vi "走到地.vi"(0 "房子數量":dbl, 1 "自己的地?":bool, 2 "旅館數量":dbl, 3 "編號":dbl, 4 "走到人財產":dbl) -> (5 "走到人-?":dbl, 6 "蓋第幾棟":dbl, 7 "地主+?":dbl, 8 "破產?":bool)   [LabVIEW 2014]
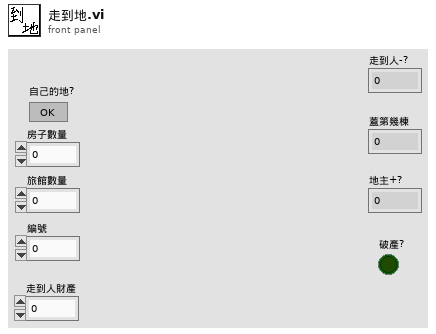
[diagram p1: front panel]
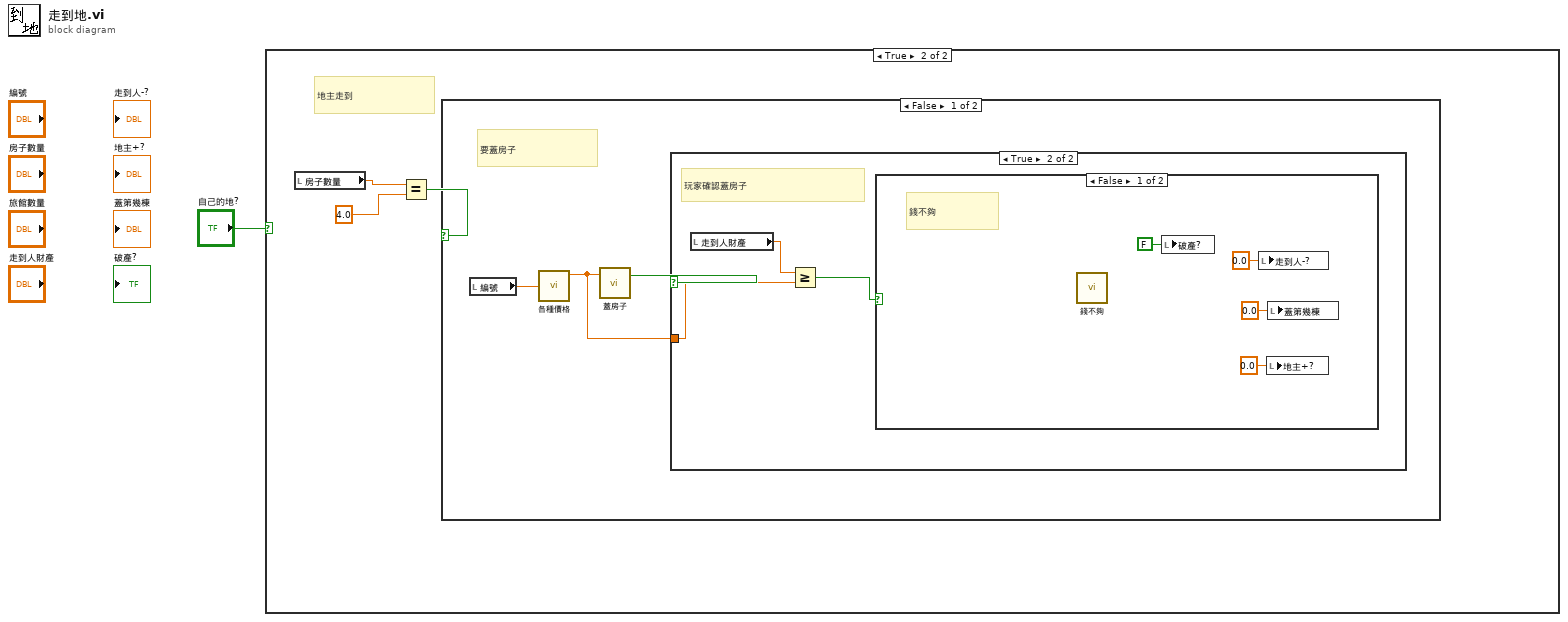
[diagram p0: block diagram]
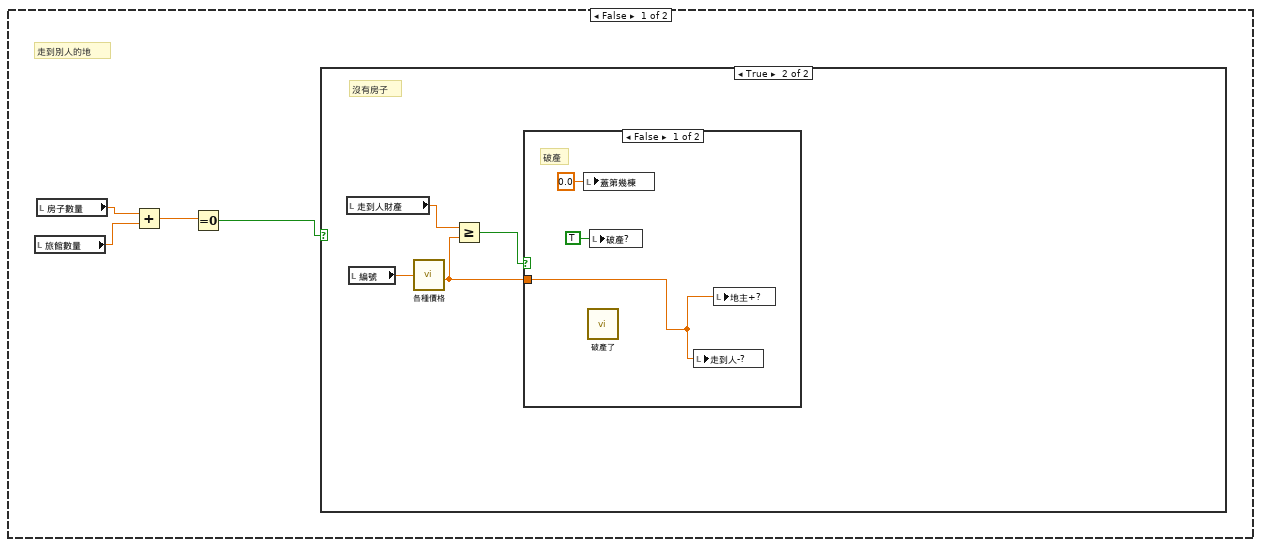
[diagram p2: hidden frame]
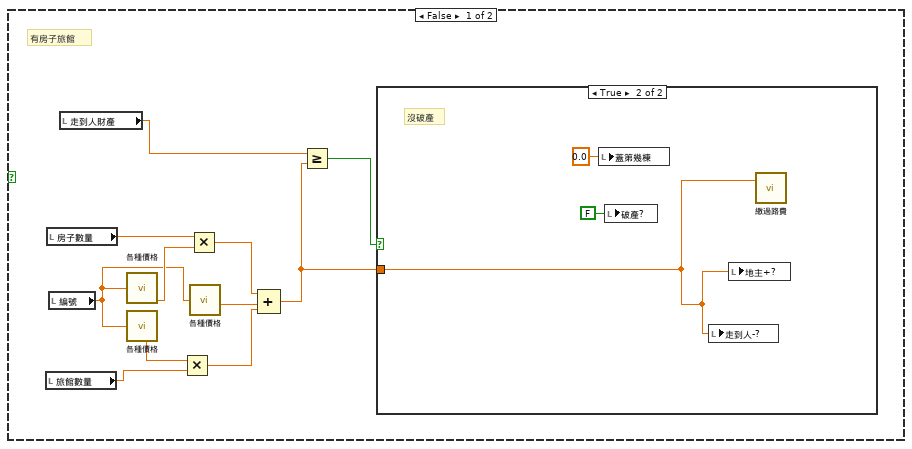
[diagram p3: hidden frame]
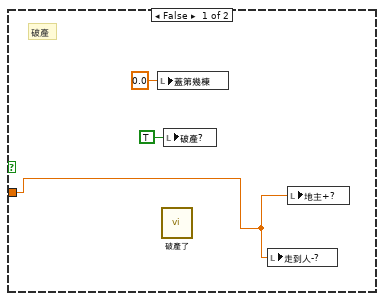
[diagram p4: hidden frame]
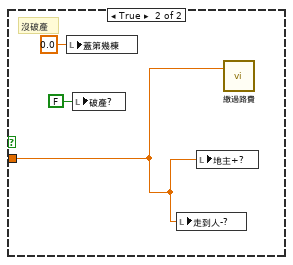
[diagram p5: hidden frame]
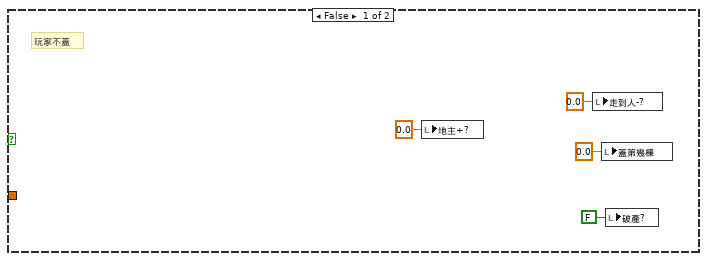
[diagram p6: hidden frame]
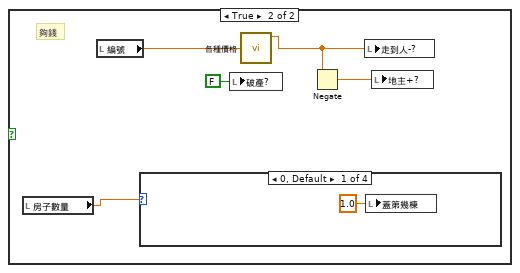
[diagram p7: hidden frame]
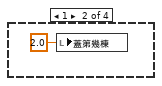
[diagram p8: hidden frame]
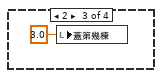
[diagram p9: hidden frame]
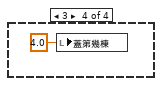
[diagram p10: hidden frame]
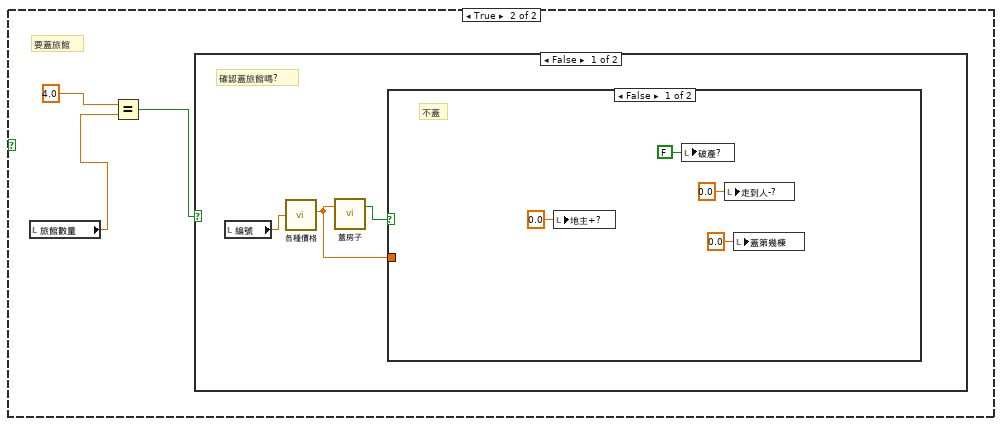
[diagram p11: hidden frame]
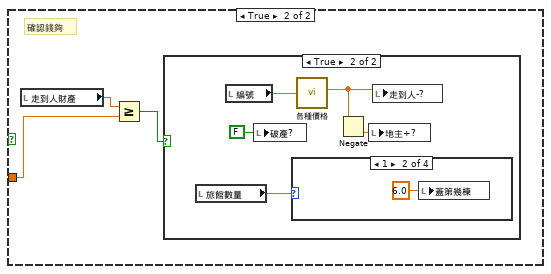
[diagram p12: hidden frame]
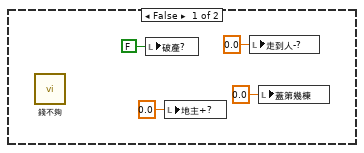
[diagram p13: hidden frame]
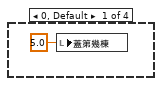
[diagram p14: hidden frame]
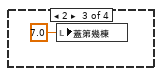
[diagram p15: hidden frame]
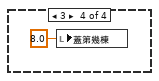
[diagram p16: hidden frame]
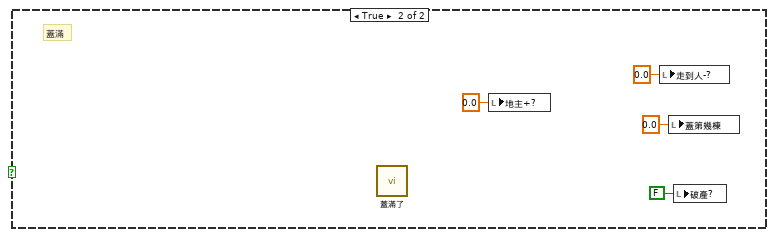
[diagram p17: hidden frame]
diagram:
  n1 = case shown="True" "自己的地?" {
    frame False {
      # "走到別人的地"
      n2 = local read "旅館數量"() -> (w4:dbl)
      n3 = local read "房子數量"() -> (w5:dbl)
      n4 = Add(x=w5, y=w4) -> (x+y=w3:dbl)
      n5 = Equal To 0?(x=w3) -> (x = 0?=w2:bool)
      n6 = case shown="True" w2 {
        frame False {
          # "有房子旅館"
          n7 = local read "旅館數量"() -> (w13:dbl)
          n8 = local read "房子數量"() -> (w16:dbl)
          n9 = local read "編號"() -> (w9:dbl)
          n10 = local read "走到人財產"() -> (w12:dbl)
          n11 = call "各種價格.vi"("Numeric"=w9) -> ("1房子費"=w15:dbl)  [unwired: 4 in, 5 out]
          n12 = call "各種價格.vi"("Numeric"=w9) -> ("1旅館費"=w14:dbl)  [unwired: 4 in, 5 out]
          n13 = Multiply(x=w14, y=w13) -> (x*y=w6:dbl)
          n14 = Multiply(x=w16, y=w15) -> (x*y=w7:dbl)
          n15 = call "各種價格.vi"("Numeric"=w9) -> ("空地費"=w8:dbl)  [unwired: 4 in, 5 out]
          n16 = Compound Arithmetic op=ADD(w7, w8, w6) -> (w10:dbl)
          n17 = Greater Or Equal?(x=w12, y=w10) -> (x >= y?=w11:bool)
          n18 = case shown="True" w11 {
            tunnel: w10 -> [w17 w20]
            frame False {
              # "破產"
              n19 = local write "蓋第幾棟"(0.0 ("蓋第幾棟")) -> ()
              n20 = call "破產了.vi"() -> ()  [unwired: 4 in]
              n21 = local write "破產?"(TRUE ("破產?")) -> ()
              n22 = local write "走到人-?"(w17) -> ()
              n23 = local write "地主+?"(w17) -> ()
            }
            frame True {
              # "沒破產"
              n24 = local write "蓋第幾棟"(0.0 ("蓋第幾棟")) -> ()
              n25 = local write "破產?"(FALSE ("破產?")) -> ()
              n26 = local write "走到人-?"(w20) -> ()
              n27 = local write "地主+?"(w20) -> ()
              n28 = call "繳過路費.vi"("過路費"=w20) -> ()  [unwired: 3 in]
            }
          }
        }
        frame True {
          # "沒有房子"
          n29 = local read "走到人財產"() -> (w25:dbl)
          n30 = local read "編號"() -> (w26:dbl)
          n31 = call "各種價格.vi"("Numeric"=w26) -> ("空地費"=w23:dbl)  [unwired: 4 in, 5 out]
          n32 = Greater Or Equal?(x=w25, y=w23) -> (x >= y?=w24:bool)
          n33 = case shown="False" w24 {
            tunnel: w23 -> [w27 w30]
            frame False {
              # "破產"
              n34 = local write "蓋第幾棟"(0.0 ("蓋第幾棟")) -> ()
              n35 = call "破產了.vi"() -> ()  [unwired: 4 in]
              n36 = local write "破產?"(TRUE ("破產?")) -> ()
              n37 = local write "走到人-?"(w27) -> ()
              n38 = local write "地主+?"(w27) -> ()
            }
            frame True {
              # "沒破產"
              n39 = local write "蓋第幾棟"(0.0 ("蓋第幾棟")) -> ()
              n40 = local write "破產?"(FALSE ("破產?")) -> ()
              n41 = local write "走到人-?"(w30) -> ()
              n42 = local write "地主+?"(w30) -> ()
              n43 = call "繳過路費.vi"("過路費"=w30) -> ()  [unwired: 3 in]
            }
          }
        }
      }
    }
    frame True {
      # "地主走到"
      n44 = local read "房子數量"() -> (w35:dbl)
      n45 = Equal?(x=w35, y=4.0) -> (x = y?=w33:bool)
      n46 = case shown="False" w33 {
        frame False {
          # "要蓋房子"
          n47 = local read "編號"() -> (w38:dbl)
          n48 = call "各種價格.vi"("Numeric"=w38) -> ("蓋房子"=w36:dbl)  [unwired: 4 in, 5 out]
          n49 = call "蓋房子.vi"("花費金額"=w36) -> ("確定 2"=w37:bool)  [unwired: 2 in]
          n50 = case shown="True" w37 {
            tunnel: w36 -> [_ w44]
            frame False {
              # "玩家不蓋"
              n51 = local write "地主+?"(0.0 ("地主+?")) -> ()
              n52 = local write "走到人-?"(0.0 ("走到人-?")) -> ()
              n53 = local write "蓋第幾棟"(0.0 ("蓋第幾棟")) -> ()
              n54 = local write "破產?"(FALSE ("破產?")) -> ()
            }
            frame True {
              # "玩家確認蓋房子"
              n55 = local read "走到人財產"() -> (w45:dbl)
              n56 = Greater Or Equal?(x=w45, y=w44) -> (x >= y?=w43:bool)
              n57 = case shown="False" w43 {
                frame False {
                  # "錢不夠"
                  n58 = call "錢不夠.vi"() -> ()  [unwired: 4 in]
                  n59 = local write "破產?"(FALSE ("破產?")) -> ()
                  n60 = local write "走到人-?"(0.0 ("走到人-?")) -> ()
                  n61 = local write "地主+?"(0.0 ("地主+?")) -> ()
                  n62 = local write "蓋第幾棟"(0.0 ("蓋第幾棟")) -> ()
                }
                frame True {
                  # "夠錢"
                  n63 = local read "房子數量"() -> (w53:dbl)
                  n64 = local read "編號"() -> (w54:dbl)
                  n65 = case shown="0, Default" w53 {
                    frame 0, Default {
                      n66 = local write "蓋第幾棟"(1.0 ("蓋第幾棟")) -> ()
                    }
                    frame 1 {
                      n67 = local write "蓋第幾棟"(2.0 ("蓋第幾棟")) -> ()
                    }
                    frame 2 {
                      n68 = local write "蓋第幾棟"(3.0 ("蓋第幾棟")) -> ()
                    }
                    frame 3 {
                      n69 = local write "蓋第幾棟"(4.0 ("蓋第幾棟")) -> ()
                    }
                  }
                  n70 = local write "破產?"(FALSE ("破產?")) -> ()
                  n71 = call "各種價格.vi"("Numeric"=w54) -> ("蓋房子"=w51:dbl)  [unwired: 4 in, 5 out]
                  n72 = Negate(x=w51) -> (-x=w50:dbl)
                  n73 = local write "走到人-?"(w51) -> ()
                  n74 = local write "地主+?"(w50) -> ()
                }
              }
            }
          }
        }
        frame True {
          # "要蓋旅館"
          n75 = local read "旅館數量"() -> (w60:dbl)
          n76 = Equal?(x=4.0 ("y"), y=w60) -> (x = y?=w59:bool)
          n77 = case shown="False" w59 {
            frame False {
              # "確認蓋旅館嗎?"
              n78 = local read "編號"() -> (w64:dbl)
              n79 = call "各種價格.vi"("Numeric"=w64) -> ("蓋旅館"=w62:dbl)  [unwired: 4 in, 5 out]
              n80 = call "蓋房子.vi"("花費金額"=w62) -> ("確定 2"=w63:bool)  [unwired: 2 in]
              n81 = case shown="False" w63 {
                tunnel: w62 -> [_ w70]
                frame False {
                  # "不蓋"
                  n82 = local write "地主+?"(0.0 ("地主+?")) -> ()
                  n83 = local write "破產?"(FALSE ("破產?")) -> ()
                  n84 = local write "走到人-?"(0.0 ("走到人-?")) -> ()
                  n85 = local write "蓋第幾棟"(0.0 ("蓋第幾棟")) -> ()
                }
                frame True {
                  # "確認錢夠"
                  n86 = local read "走到人財產"() -> (w71:dbl)
                  n87 = Greater Or Equal?(x=w71, y=w70) -> (x >= y?=w69:bool)
                  n88 = case shown="True" w69 {
                    frame False {
                      n89 = call "錢不夠.vi"() -> ()  [unwired: 4 in]
                      n90 = local write "破產?"(FALSE ("破產?")) -> ()
                      n91 = local write "地主+?"(0.0 ("地主+?")) -> ()
                      n92 = local write "走到人-?"(0.0 ("走到人-?")) -> ()
                      n93 = local write "蓋第幾棟"(0.0 ("蓋第幾棟")) -> ()
                    }
                    frame True {
                      n94 = local read "旅館數量"() -> (w79:dbl)
                      n95 = local read "編號"() -> (w80:dbl)
                      n96 = local write "破產?"(FALSE ("破產?")) -> ()
                      n97 = case shown="1" w79 {
                        frame 0, Default {
                          n98 = local write "蓋第幾棟"(5.0 ("蓋第幾棟")) -> ()
                        }
                        frame 1 {
                          n99 = local write "蓋第幾棟"(6.0 ("蓋第幾棟")) -> ()
                        }
                        frame 2 {
                          n100 = local write "蓋第幾棟"(7.0 ("蓋第幾棟")) -> ()
                        }
                        frame 3 {
                          n101 = local write "蓋第幾棟"(8.0 ("蓋第幾棟")) -> ()
                        }
                      }
                      n102 = call "各種價格.vi"("Numeric"=w80) -> ("蓋旅館"=w77:dbl)  [unwired: 4 in, 5 out]
                      n103 = Negate(x=w77) -> (-x=w76:dbl)
                      n104 = local write "地主+?"(w76) -> ()
                      n105 = local write "走到人-?"(w77) -> ()
                    }
                  }
                }
              }
            }
            frame True {
              # "蓋滿"
              n106 = call "蓋滿了.vi"() -> ()  [unwired: 4 in]
              n107 = local write "地主+?"(0.0 ("地主+?")) -> ()
              n108 = local write "走到人-?"(0.0 ("走到人-?")) -> ()
              n109 = local write "蓋第幾棟"(0.0 ("蓋第幾棟")) -> ()
              n110 = local write "破產?"(FALSE ("破產?")) -> ()
            }
          }
        }
      }
    }
  }
